vi "ConfigureVibrationAnalysis.vi"(8 "error in (no error)":errorcluster) -> (0 "error out":errorcluster, 2 "register trends":T1[](array[typedef]), 3 "analysis config":T3, 5 "all config found?":bool)   [LabVIEW 2015]
uses:
  <vilib>/addons/InsightCM/Devices/Shared/VibrationAnalysisLoop/controls/Config.ctl
  <vilib>/addons/InsightCM/Devices/Shared/VibrationAnalysisLoop/controls/Group.ctl
  <vilib>/addons/InsightCM/Utilities/Analysis/Shared/controls/Channel.ctl
  <vilib>/addons/InsightCM/Utilities/Analysis/Shared/controls/Feature.ctl
  <vilib>/addons/InsightCM/Utilities/Analysis/Shared/controls/AmplitudeScale.ctl
  <vilib>/addons/InsightCM/Utilities/ChannelStatus/controls/RangeParams.ctl
  <vilib>/addons/InsightCM/Devices/Shared/TdmsCreator/controls/RegisterTrendTdmsPropertiesRoutedMessage.ctl
  <vilib>/addons/InsightCM/Devices/Shared/TdmsCreator/controls/Trend.ctl
  <vilib>/addons/InsightCM/Utilities/Analysis/Shared/AnalysisHelper.lvlib
  <vilib>/addons/InsightCM/Utilities/GlobalConfiguration/GlobalConfiguration.lvlib
  <vilib>/addons/InsightCM/Utilities/DeviceModelHelpers/DeviceModelHelpers.lvlib
  <vilib>/addons/InsightCM/Devices/Shared/VibrationAnalysisLoop/VibrationAnalysis.lvlib
  <vilib>/addons/InsightCM/Utilities/ChannelStatus/ChannelStatus.lvlib
  <vilib>/addons/InsightCM/Devices/Shared/VibrationVirtualChannel/VibrationVirtualChannel.lvlib
  <vilib>/addons/InsightCM/Utilities/PropertyHelpers/PropertyHelpers.lvlib
  <vilib>/addons/InsightCM/Devices/Shared/TdmsCreator/TdmsCreator.lvlib
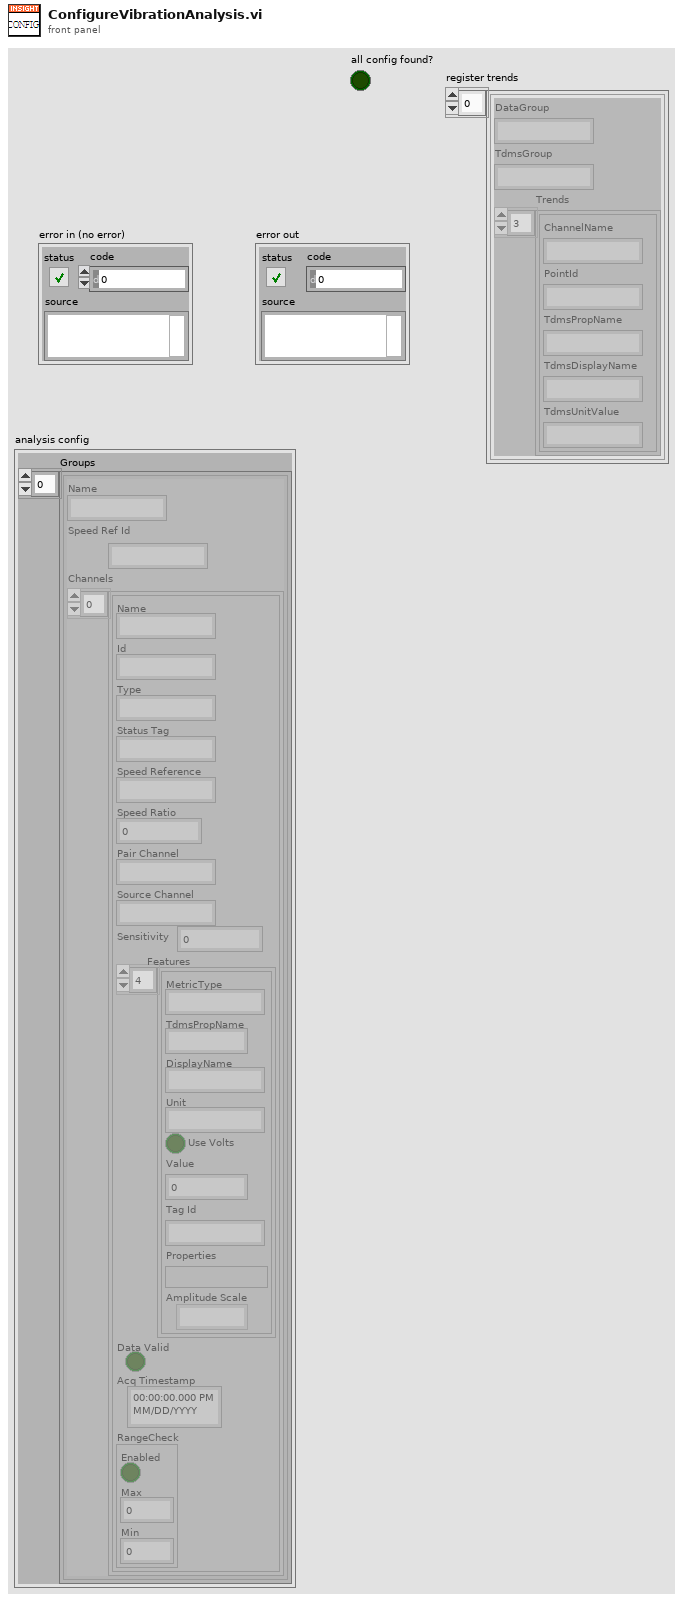
[diagram p1: front panel]
types:
  T1 = typedef "TdmsCreator.lvlib/RegisterTrendTdmsPropertiesRoutedMessage.ctl" = cluster{"DataGroup":string, "TdmsGroup":string, "Trends":T2[]}
  T2 = typedef "TdmsCreator.lvlib/Trend.ctl" = cluster{"ChannelName":string, "PointId":string, "TdmsPropName":string, "TdmsDisplayName":string, "TdmsUnitValue":string}
  T3 = typedef "VibrationAnalysis.lvlib/Config.ctl" = cluster{"Groups":T4[]}
  T4 = typedef "VibrationAnalysis.lvlib/Group.ctl" = cluster{"Name":string, "Speed Ref Id":string, "Channels":T5[]}
  T5 = typedef "AnalysisHelper.lvlib/Channel.ctl" = cluster{"Name":string, "Id":string, "Type":string, "Status Tag":string, "Speed Reference":string, "Speed Ratio":dbl, "Pair Channel":string, "Source Channel":string, "Sensitivity":dbl, "Features":T6[], "Data Valid":bool, "Acq Timestamp":timestamp, "RangeCheck":T8}
  T6 = typedef "AnalysisHelper.lvlib/Feature.ctl" = cluster{"MetricType":string, "TdmsPropName":string, "DisplayName":string, "Unit":string, "Use Volts":bool, "Value":dbl, "Tag Id":string, "Properties":variant, "Amplitude Scale":T7}
  T7 = typedef "AnalysisHelper.lvlib/AmplitudeScale.ctl" = enum16{"rms", "peak", "pk-pk"}
  T8 = typedef "ChannelStatus.lvlib/RangeParams.ctl" = cluster{"Enabled":bool, "Max":dbl, "Min":dbl}
  T9 = typedef "DeviceModel.ctl" = cluster{"Device":T10, "Channels":T16[], "Tags":T18[]}
  T10 = typedef "Device.ctl" = cluster{"Id":string, "Name":string, "DeviceType":string, "HardwareName":string, "IpAddress":string, "HardwareInfo":T11[], "ApplicationType":string, "ApplicationVersion":string, "EquipmentIds":string[], "ConfigurationVersion":string, "Properties":T11[], "DataGroups":T12[]}
  T11 = typedef "KeyValuePair.ctl" = cluster{"Key":string, "Value":string}
  T12 = typedef "DataGroup.ctl" = cluster{"Name":string, "OperatingStates":T13[], "Properties":T11[], "EquipmentIds":string[]}
  T13 = typedef "OperatingState.ctl" = cluster{"Name":string, "Properties":T11[], "Triggers":T14[]}
  T14 = typedef "Trigger.ctl" = cluster{"Type":string, "Expression":string, "Conditions":T15[]}
  T15 = typedef "Condition.ctl" = cluster{"Source":string, "Type":string, "Operator":string, "CompareTo":string, "DwellSeconds":dbl}
  T16 = typedef "Channel.ctl" = cluster{"Id":string, "DeviceId":string, "Name":string, "ChannelType":string, "HardwareKey":string, "HardwareChannel":string, "DataGroup":string, "Keywords":string[], "EquipmentIds":string[], "Properties":T11[], "Metrics":T17[]}
  T17 = typedef "MetricModel.ctl" = cluster{"Id":string, "MetricDefinitionInstanceId":string, "Properties":T11[]}
  T18 = typedef "Tag.ctl" = cluster{"Id":string, "Path":string, "Name":string, "Datatype":string, "Props":T11[], "Keywords":string[]}
  T19 = typedef "SectionKeyValues.ctl" = cluster{"Section":string, "KeyValues":T11[]}
  T20 = typedef "MetricDefinitionInstance.ctl" = cluster{"Id":string, "MetricType":string, "Name":string, "Properties":T11[], "MetricChannelTypes":T21[]}
  T21 = typedef "MetricChannelType.ctl" = cluster{"ChannelType":string, "Required":bool, "Properties":T11[]}
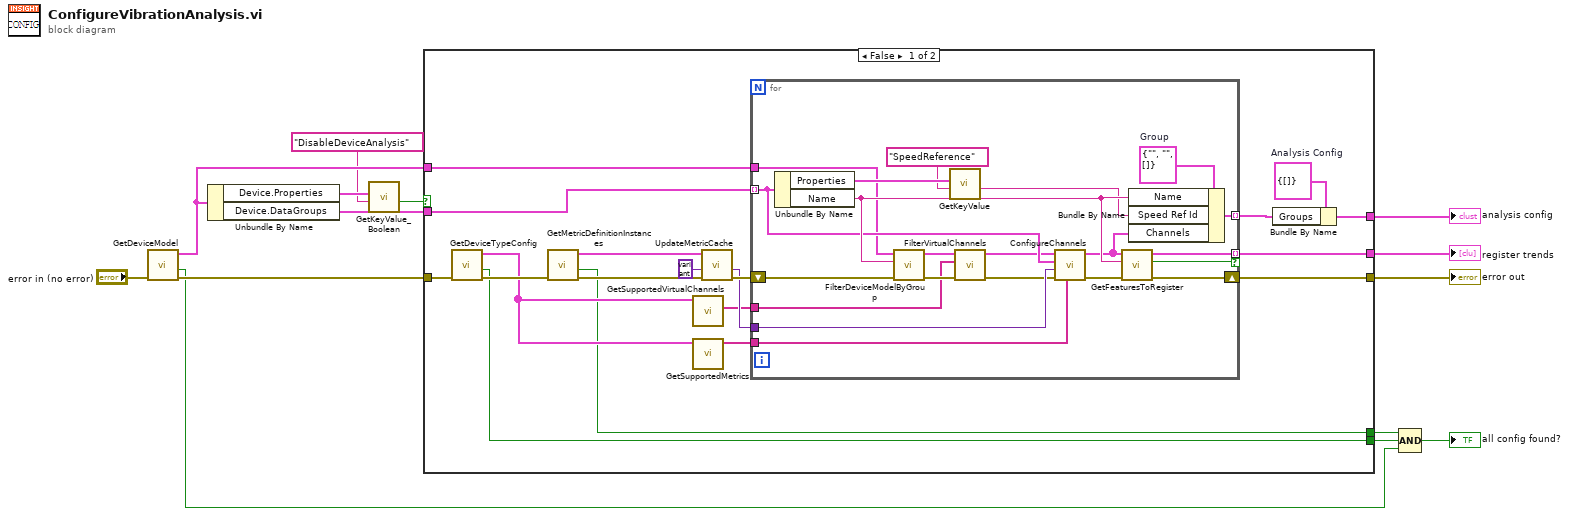
[diagram p0: block diagram]
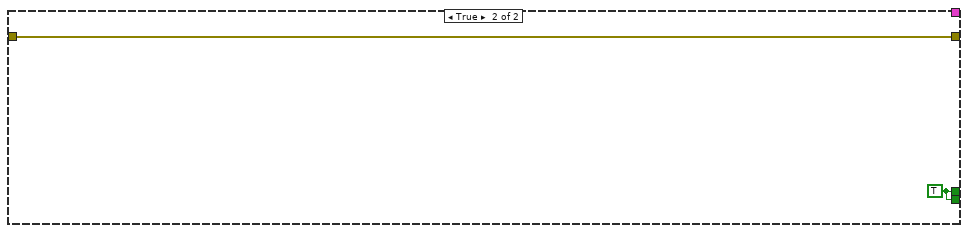
[diagram p2: hidden frame]
diagram:
  n1 = call <vilib>:"GetDeviceModel.vi"("error in (no error)"="error in (no error)") -> ("error out"=w9:errorcluster, "found"=w4:bool, "device model"=w8:T9)  [unwired: 8 in]
  n2 = Unbundle By Name(w8) -> ("Device.Properties"=w7:T11[], "Device.DataGroups"=w14:T12[])
  n3 = call <vilib>:"GetKeyValue_Boolean.vi"("key"="DisableDeviceAnalysis", "key value pairs"=w7) -> ("value"=w5:bool)  [unwired: 7 in, 2 out]
  n4 = case shown="False" w5 {
    tunnel: w14 -> [w28 _]
    tunnel: [w27 w56] -> w13
    tunnel: [w26 _] -> w12
    tunnel: [w24 _] -> w11
    tunnel: w9 -> [w18 w56]
    tunnel: w8 -> [w17 _]
    tunnel: [w16 w55] -> w3
    tunnel: [w15 w55] -> w2
    frame False {
      w25 = T3 {"Groups"=[]}  # Analysis Config
      n5 = call <vilib>:"GetDeviceTypeConfig.vi"("error in (no error)"=w18) -> ("error out"=w22:errorcluster, "found"=w15:bool, "key values"=w20:T19[])  [unwired: 8 in]
      n6 = call <vilib>:"GetMetricDefinitionInstances.vi"("error in (no error)"=w22) -> ("error out"=w33:errorcluster, "found"=w16:bool, "metrics"=w31:T20[])  [unwired: 8 in]
      n7 = call <vilib>:"GetSupportedVirtualChannels.vi"("key values"=w20) -> ("not supported virtual channels"=w19:string[])  [unwired: 9 in, 1 out]
      n8 = call <vilib>:"GetSupportedMetrics.vi"("key values"=w20) -> ("supported metrics"=w21:string[])  [unwired: 10 in]
      n9 = call "UpdateMetricCache.vi"("error in (no error)"=w33, "Metrics"=variant, "MetricDefinitionInstances"=w31) -> ("error out"=w32:errorcluster, "Metrics out"=w30:variant)  [unwired: 7 in]
      n10 = for {
        tunnel: w30 -> [w54]
        tunnel: w17 -> [w35]
        shift-right: [w51] -> w27
        shift-left: w32 -> [w52]
        tunnel: [w53] -> w23 mode=indexing
        tunnel: w28 -> [w46] mode=indexing
        tunnel: [w50] -> w26 mode=indexing if=w49
        tunnel: w21 -> [w45]
        tunnel: w19 -> [w38]
        w47 = T4 {"Name"="", "Speed Ref Id"="", "Channels"=[]}  # Group
        n11 = Unbundle By Name(w46) -> ("Properties"=w37:T11[], "Name"=w48:string)
        n12 = call <vilib>:"FilterDeviceModelByGroup.vi"("error in (no error)"=w52, "group"=w48, "device model"=w35) -> ("error out"=w39:errorcluster, "device model (channels filtered by group)"=w41:T9)  [unwired: 7 in]
        n13 = call <vilib>:"GetKeyValue.vi"("key"="SpeedReference", "key value pairs"=w37) -> ("value"=w34:string)  [unwired: 7 in, 2 out]
        n14 = call <vilib>:"FilterVirtualChannels.vi"("error in (no error)"=w39, "not supported virtual channels"=w38, "device model"=w41) -> ("error out"=w40:errorcluster, "device model (unsupported virtual channels filtered out)"=w42:T9)  [unwired: 7 in]
        n15 = call <vilib>:"ConfigureChannels.vi"("supported metrics"=w45, "error in (no error)"=w40, "metric cache"=w54, "group"=w46, "device"=w42) -> ("error out"=w43:errorcluster, "channels"=w44:T5[])  [unwired: 5 in]
        n16 = call <vilib>:"GetFeaturesToRegister.vi"("error in (no error)"=w43, "group"=w48, "channels"=w44) -> ("error out"=w51:errorcluster, "atleast one"=w49:bool, "register trend"=w50:T1)  [unwired: 6 in]
        n17 = Bundle By Name(cluster=w47, "Name"=w48, "Speed Ref Id"=w34, "Channels"=w44) -> (w53:T4)
      }
      n18 = Bundle By Name(cluster=w25, "Groups"=w23) -> (w24:T3)
    }
    frame True {
      w55 = TRUE ("found")
    }
  }
  "error out" <- w13
  "analysis config" <- w11
  "register trends" <- w12
  n19 = Compound Arithmetic op=AND(w3, w2, w4) -> (→"all config found?":bool)
